vi "Remove DC Offset through Scaling.vi"(1 "unscaled array":dbl[](array[numeric])) -> (0 "scaled array":dbl[](array[numeric]))   [LabVIEW 2010]
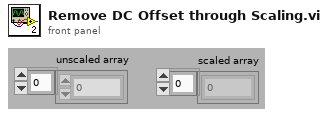
[diagram p1: front panel]
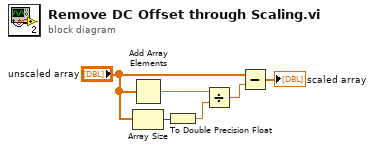
[diagram p0: block diagram]
diagram:
  n1 = Add Array Elements(numeric array="unscaled array") -> (sum=w4:dbl)
  n2 = Array Size(array="unscaled array") -> (size(s)=w6:i32)
  n3 = To Double Precision Float(number=w6) -> (double precision float=w5:dbl)
  n4 = Divide(x=w4, y=w5) -> (x/y=w3:dbl)
  n5 = Subtract(x="unscaled array", y=w3) -> (x-y=→"scaled array":dbl[])
